vi "Get Icon Path.vi"(8 "Error In":errorcluster, 11 "Context":refnum<k7>) -> (0 "Error Out":errorcluster, 2 "Path":path, 3 "Found?":bool)   [LabVIEW 2021, in "Seq Edit Quick Drop.lvlib"]
uses:
  Seq Edit Quick Drop.lvlib
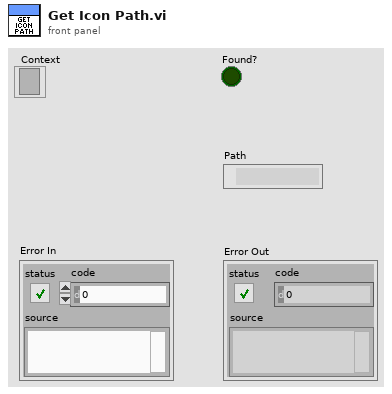
[diagram p1: front panel]
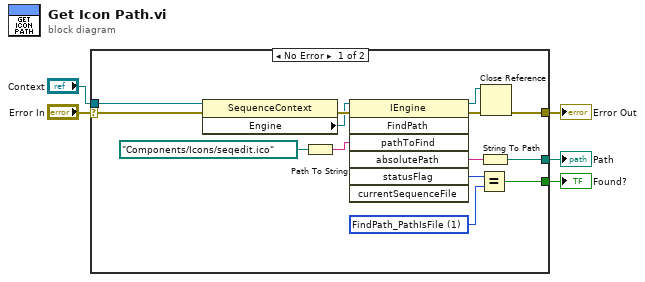
[diagram p0: block diagram]
diagram:
  n1 = case shown="No Error" "Error In" {
    selector: "Error In" -> [w8 w20]
    tunnel: "Context" -> [w18 _]
    tunnel: [w9 w20] -> w4
    tunnel: [w7 _] -> w2
    tunnel: [w6 _] -> w1
    frame No Error {
      w11 = 1 items=["FindPath_PathIsFile"=1, "FindPath_PathIsDir"=2, "FindPath_PathNotFound"=3, "FindPath_PathNotValid"=4] ("statusFlag")
      n2 = property class="SequenceContext"(reference=w18, error in=w8) -> (error out=w19:errorcluster, "Engine"=w17:refnum<k7>)  [unwired: 1 out]
      n3 = Path To String(path=path "Components/Icons/seqedit.ico" ("name or relative path")) -> (string=w15:string)
      n4 = invoke class="IEngine" method="FindPath"(reference=w17, error in=w19, "pathToFind"=w15) -> (reference out=w13:refnum<k7>, error out=w14:errorcluster, "absolutePath"=w12:string, "statusFlag"=w10:i32)  [unwired: 4 in, 3 out]
      n5 = Equal?(x=w10, y=w11) -> (x = y?=w6:bool)
      n6 = String To Path(string=w12) -> (path=w7:path)
      n7 = Close Reference(reference=w13, error in (no error)=w14) -> (error out=w9:errorcluster)
    }
    frame Error {
    }
  }
  "Error Out" <- w4
  "Found?" <- w1
  "Path" <- w2
